vi "Init Task.vi"(6 "line grouping":i32(ring) items=["one channel for each line", "one channel for all lines"], 7 "counter":tag, 8 "error in (no error)":errorcluster, 9 "name":string, 10 "physical channels":tag, 11 "DAQmxTask in":refnum<class "DAQmxTask.lvclass">) -> (0 "error out":errorcluster, 3 "DAQmxTask out":refnum<class "DAQmxTask.lvclass">)   [LabVIEW 2015, in "DAQmxTask.lvclass"]
uses:
  DAQmxTask.lvclass
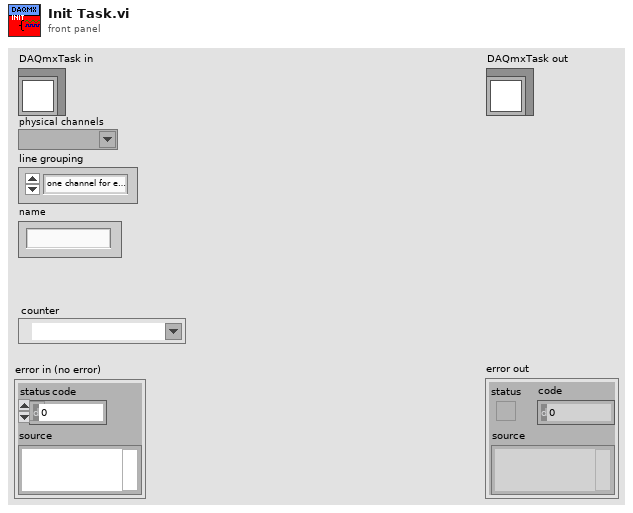
[diagram p1: front panel]
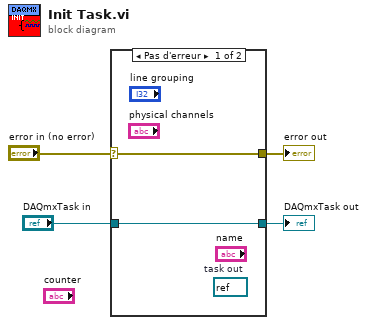
[diagram p0: block diagram]
diagram:
  n1 = case shown="Pas d'erreur" "error in (no error)" {
    selector: "error in (no error)" -> [w5 w8]
    tunnel: [w5 w8] -> w3
    tunnel: [w6 w7] -> w1
    tunnel: "DAQmxTask in" -> [w6 w7]
    frame No Error {
      (unwired) refnum<k21> refnum  # task out
    }
    frame Error {
    }
  }
  "error out" <- w3
  "DAQmxTask out" <- w1
